vi "HumanDriveButtonBoxSourceClimbProcessor.vi"(6 "Processor":bool, 7 "Climb":bool, 8 "LeftSourceLeft":bool, 9 "LeftSourceRight":bool, 10 "RightSourceLeft":bool, 11 "RightSourceRight":bool) -> (3 "DriveTraj":bool)   [LabVIEW 2023]
uses:
  HumanGlobal.vi
  <vilib>/Rock Robotics/WPI/ThirdParty/JAS_Junk/TrajLib/Trajectory_Library.lvlib
  HumanBoxSourceClimbProcessorENUM.ctl
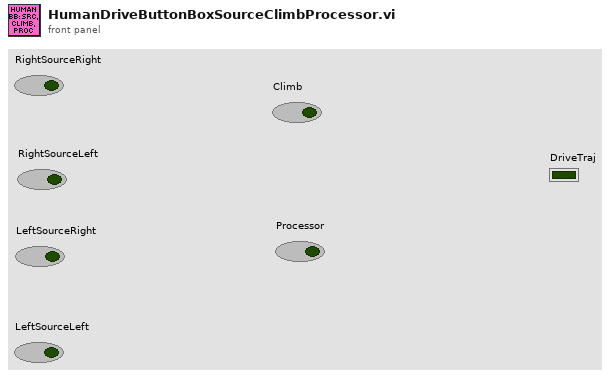
[diagram p1: front panel]
types:
  T1 = typedef "HumanBoxSourceClimbProcessorENUM.ctl" = enum16{"NoTraj", "RightSourceRight", "RightSourceLeft", "LeftSourceRight", "LeftSourceLeft", "Climb", "Processor"}
  T2 = typedef "WPI_DriverStationAllianceInfo.ctl" = enum16{"Red", "Blue", "Invalid"}
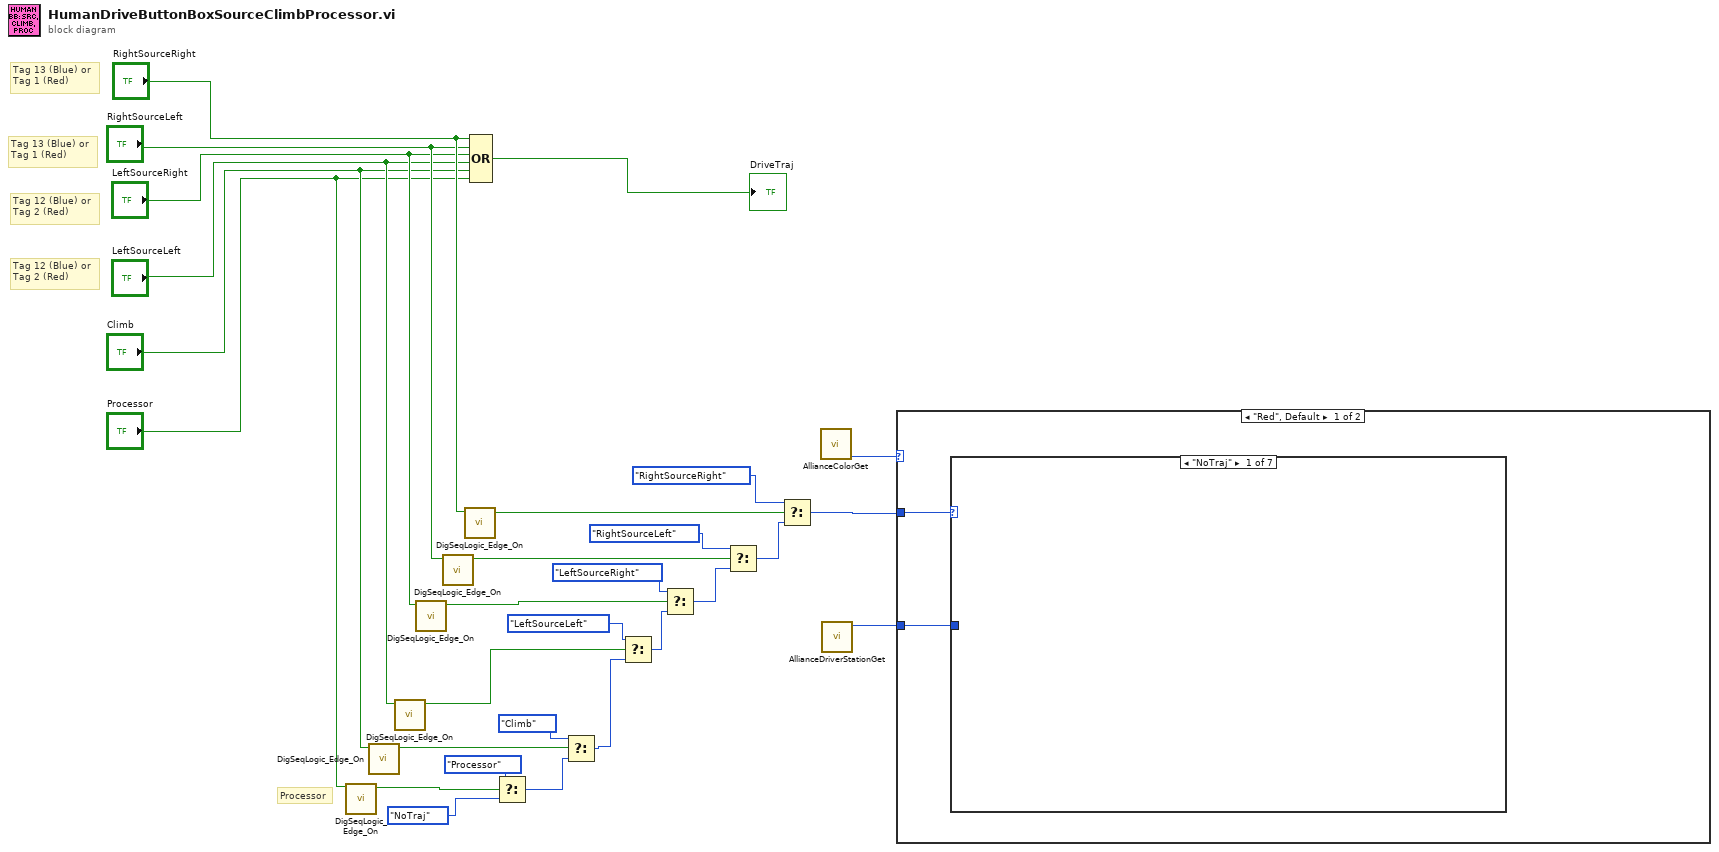
[diagram p0: block diagram]
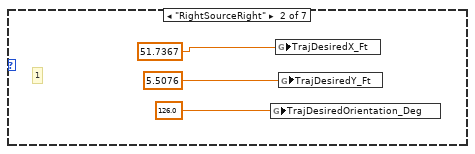
[diagram p2: hidden frame]
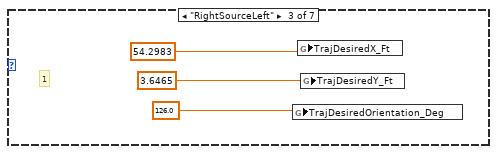
[diagram p3: hidden frame]
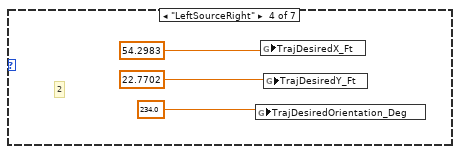
[diagram p4: hidden frame]
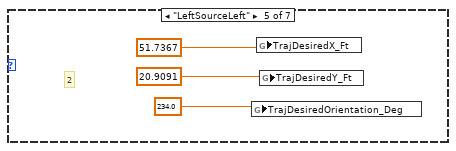
[diagram p5: hidden frame]
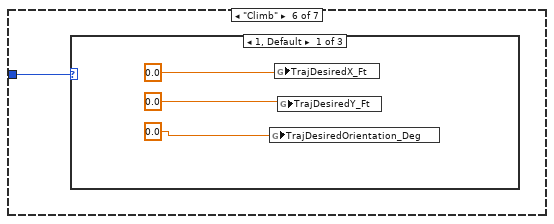
[diagram p6: hidden frame]
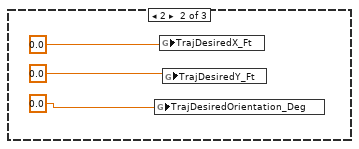
[diagram p7: hidden frame]
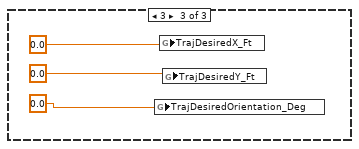
[diagram p8: hidden frame]
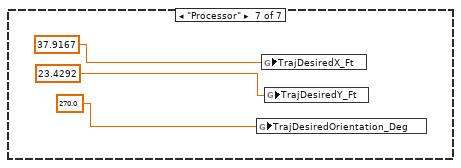
[diagram p9: hidden frame]
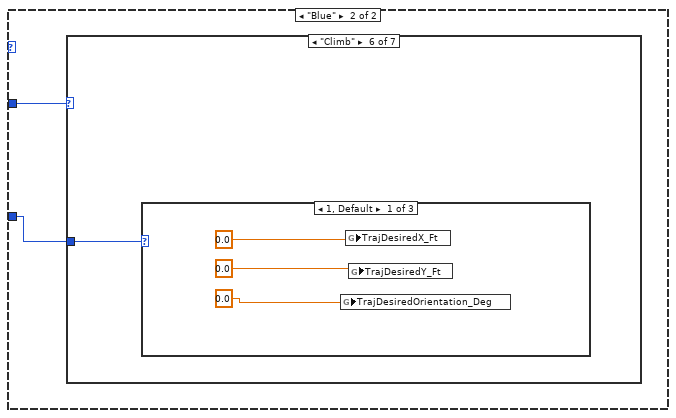
[diagram p10: hidden frame]
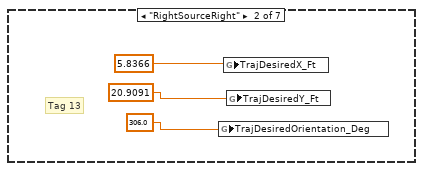
[diagram p12: hidden frame]
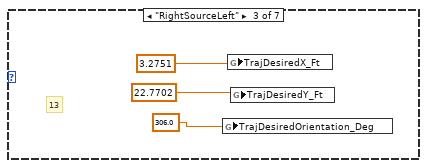
[diagram p13: hidden frame]
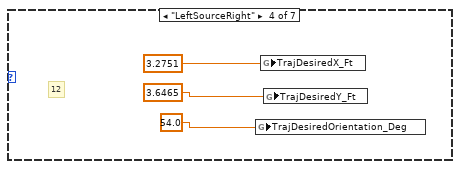
[diagram p14: hidden frame]
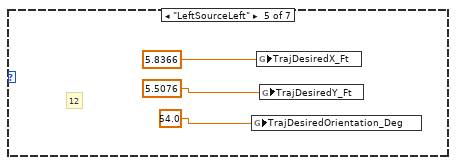
[diagram p15: hidden frame]
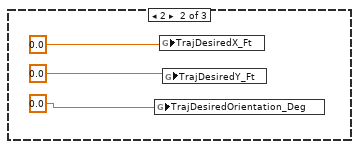
[diagram p16: hidden frame]
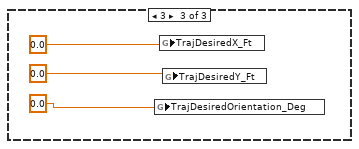
[diagram p17: hidden frame]
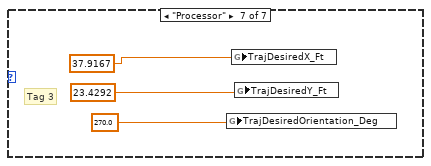
[diagram p18: hidden frame]
diagram:
  # "Tag 13 (Blue) or \nTag 1 (Red)"
  # "Tag 13 (Blue) or \nTag 1 (Red)"
  # "Tag 12 (Blue) or \nTag 2 (Red)"
  # "Tag 12 (Blue) or \nTag 2 (Red)"
  # "Processor"
  n1 = call <vilib>:"DigSeqLogic_Edge_On.vi"("Input"="Processor") -> ("On Edge"=w21:bool)  [unwired: 10 in]
  n2 = call <vilib>:"DigSeqLogic_Edge_On.vi"("Input"="Climb") -> ("On Edge"=w15:bool)  [unwired: 10 in]
  n3 = call <vilib>:"DigSeqLogic_Edge_On.vi"("Input"="LeftSourceLeft") -> ("On Edge"=w14:bool)  [unwired: 10 in]
  n4 = call <vilib>:"DigSeqLogic_Edge_On.vi"("Input"="LeftSourceRight") -> ("On Edge"=w13:bool)  [unwired: 10 in]
  n5 = call <vilib>:"DigSeqLogic_Edge_On.vi"("Input"="RightSourceLeft") -> ("On Edge"=w12:bool)  [unwired: 10 in]
  n6 = call <vilib>:"DigSeqLogic_Edge_On.vi"("Input"="RightSourceRight") -> ("On Edge"=w11:bool)  [unwired: 10 in]
  n7 = Compound Arithmetic op=OR("RightSourceRight", "RightSourceLeft", "LeftSourceRight", "LeftSourceLeft", "Climb", "Processor") -> (→"DriveTraj":bool)
  n8 = Select(t=HumanBoxSourceClimbProcessorENUM."Processor", s=w21, f=HumanBoxSourceClimbProcessorENUM."NoTraj") -> (s? t:f=w20:T1)
  n9 = Select(t=HumanBoxSourceClimbProcessorENUM."Climb", s=w15, f=w20) -> (s? t:f=w19:T1)
  n10 = Select(t=HumanBoxSourceClimbProcessorENUM."LeftSourceLeft", s=w14, f=w19) -> (s? t:f=w18:T1)
  n11 = Select(t=HumanBoxSourceClimbProcessorENUM."LeftSourceRight", s=w13, f=w18) -> (s? t:f=w17:T1)
  n12 = Select(t=HumanBoxSourceClimbProcessorENUM."RightSourceLeft", s=w12, f=w17) -> (s? t:f=w16:T1)
  n13 = Select(t=HumanBoxSourceClimbProcessorENUM."RightSourceRight", s=w11, f=w16) -> (s? t:f=w3:T1)
  n14 = call "AllianceColorGet.vi"() -> ("AllianceColor"=w2:T2)  [unwired: 11 in]
  n15 = call "AllianceDriverStationGet.vi"() -> ("Position"=w1:i32)  [unwired: 11 in]
  n16 = case shown="\"Red\", Default" w2 {
    tunnel: w3 -> [w30 w57]
    tunnel: w1 -> [w29 w56]
    frame "Red", Default {
      n17 = case shown="\"NoTraj\"" w30 {
        tunnel: w29 -> [_ _ _ _ _ w43 _]
        frame "NoTraj" {
        }
        frame "RightSourceRight" {
          # "1"
          n18 = global write "HumanGlobal.vi" "TrajDesiredOrientation_Deg"(126.0 ("TrajDesiredOrientation_Deg")) -> ()
          n19 = global write "HumanGlobal.vi" "TrajDesiredX_Ft"(51.7367 ("TrajDesiredX_Ft")) -> ()
          n20 = global write "HumanGlobal.vi" "TrajDesiredY_Ft"(5.5076 ("TrajDesiredY_Ft")) -> ()
        }
        frame "RightSourceLeft" {
          # "1"
          n21 = global write "HumanGlobal.vi" "TrajDesiredOrientation_Deg"(126.0 ("TrajDesiredOrientation_Deg")) -> ()
          n22 = global write "HumanGlobal.vi" "TrajDesiredX_Ft"(54.2983 ("TrajDesiredX_Ft")) -> ()
          n23 = global write "HumanGlobal.vi" "TrajDesiredY_Ft"(3.6465 ("TrajDesiredY_Ft")) -> ()
        }
        frame "LeftSourceRight" {
          # "2"
          n24 = global write "HumanGlobal.vi" "TrajDesiredOrientation_Deg"(234.0 ("TrajDesiredOrientation_Deg")) -> ()
          n25 = global write "HumanGlobal.vi" "TrajDesiredX_Ft"(54.2983 ("TrajDesiredX_Ft")) -> ()
          n26 = global write "HumanGlobal.vi" "TrajDesiredY_Ft"(22.7702 ("TrajDesiredY_Ft")) -> ()
        }
        frame "LeftSourceLeft" {
          # "2"
          n27 = global write "HumanGlobal.vi" "TrajDesiredOrientation_Deg"(234.0 ("TrajDesiredOrientation_Deg")) -> ()
          n28 = global write "HumanGlobal.vi" "TrajDesiredX_Ft"(51.7367 ("TrajDesiredX_Ft")) -> ()
          n29 = global write "HumanGlobal.vi" "TrajDesiredY_Ft"(20.9091 ("TrajDesiredY_Ft")) -> ()
        }
        frame "Climb" {
          n30 = case shown="1, Default" w43 {
            frame 1, Default {
              n31 = global write "HumanGlobal.vi" "TrajDesiredOrientation_Deg"(0.0 ("TrajDesiredOrientation_Deg")) -> ()
              n32 = global write "HumanGlobal.vi" "TrajDesiredX_Ft"(0.0 ("TrajDesiredX_Ft")) -> ()
              n33 = global write "HumanGlobal.vi" "TrajDesiredY_Ft"(0.0 ("TrajDesiredY_Ft")) -> ()
            }
            frame 2 {
              n34 = global write "HumanGlobal.vi" "TrajDesiredOrientation_Deg"(0.0 ("TrajDesiredOrientation_Deg")) -> ()
              n35 = global write "HumanGlobal.vi" "TrajDesiredX_Ft"(0.0 ("TrajDesiredX_Ft")) -> ()
              n36 = global write "HumanGlobal.vi" "TrajDesiredY_Ft"(0.0 ("TrajDesiredY_Ft")) -> ()
            }
            frame 3 {
              n37 = global write "HumanGlobal.vi" "TrajDesiredOrientation_Deg"(0.0 ("TrajDesiredOrientation_Deg")) -> ()
              n38 = global write "HumanGlobal.vi" "TrajDesiredX_Ft"(0.0 ("TrajDesiredX_Ft")) -> ()
              n39 = global write "HumanGlobal.vi" "TrajDesiredY_Ft"(0.0 ("TrajDesiredY_Ft")) -> ()
            }
          }
        }
        frame "Processor" {
          n40 = global write "HumanGlobal.vi" "TrajDesiredOrientation_Deg"(270.0 ("TrajDesiredOrientation_Deg")) -> ()
          n41 = global write "HumanGlobal.vi" "TrajDesiredX_Ft"(37.9167 ("TrajDesiredX_Ft")) -> ()
          n42 = global write "HumanGlobal.vi" "TrajDesiredY_Ft"(23.4292 ("TrajDesiredY_Ft")) -> ()
        }
      }
    }
    frame "Blue" {
      n43 = case shown="\"Climb\"" w57 {
        tunnel: w56 -> [_ _ _ _ _ w70 _]
        frame "NoTraj" {
        }
        frame "RightSourceRight" {
          # "Tag 13"
          n44 = global write "HumanGlobal.vi" "TrajDesiredOrientation_Deg"(306.0 ("TrajDesiredOrientation_Deg")) -> ()
          n45 = global write "HumanGlobal.vi" "TrajDesiredX_Ft"(5.8366 ("TrajDesiredX_Ft")) -> ()
          n46 = global write "HumanGlobal.vi" "TrajDesiredY_Ft"(20.9091 ("TrajDesiredY_Ft")) -> ()
        }
        frame "RightSourceLeft" {
          # "13"
          n47 = global write "HumanGlobal.vi" "TrajDesiredOrientation_Deg"(306.0 ("TrajDesiredOrientation_Deg")) -> ()
          n48 = global write "HumanGlobal.vi" "TrajDesiredX_Ft"(3.2751 ("TrajDesiredX_Ft")) -> ()
          n49 = global write "HumanGlobal.vi" "TrajDesiredY_Ft"(22.7702 ("TrajDesiredY_Ft")) -> ()
        }
        frame "LeftSourceRight" {
          # "12"
          n50 = global write "HumanGlobal.vi" "TrajDesiredOrientation_Deg"(54.0 ("TrajDesiredOrientation_Deg")) -> ()
          n51 = global write "HumanGlobal.vi" "TrajDesiredX_Ft"(3.2751 ("TrajDesiredX_Ft")) -> ()
          n52 = global write "HumanGlobal.vi" "TrajDesiredY_Ft"(3.6465 ("TrajDesiredY_Ft")) -> ()
        }
        frame "LeftSourceLeft" {
          # "12"
          n53 = global write "HumanGlobal.vi" "TrajDesiredOrientation_Deg"(54.0 ("TrajDesiredOrientation_Deg")) -> ()
          n54 = global write "HumanGlobal.vi" "TrajDesiredX_Ft"(5.8366 ("TrajDesiredX_Ft")) -> ()
          n55 = global write "HumanGlobal.vi" "TrajDesiredY_Ft"(5.5076 ("TrajDesiredY_Ft")) -> ()
        }
        frame "Climb" {
          n56 = case shown="1, Default" w70 {
            frame 1, Default {
              n57 = global write "HumanGlobal.vi" "TrajDesiredOrientation_Deg"(0.0 ("TrajDesiredOrientation_Deg")) -> ()
              n58 = global write "HumanGlobal.vi" "TrajDesiredX_Ft"(0.0 ("TrajDesiredX_Ft")) -> ()
              n59 = global write "HumanGlobal.vi" "TrajDesiredY_Ft"(0.0 ("TrajDesiredY_Ft")) -> ()
            }
            frame 2 {
              n60 = global write "HumanGlobal.vi" "TrajDesiredOrientation_Deg"(0.0 ("TrajDesiredOrientation_Deg")) -> ()
              n61 = global write "HumanGlobal.vi" "TrajDesiredX_Ft"(0.0 ("TrajDesiredX_Ft")) -> ()
              n62 = global write "HumanGlobal.vi" "TrajDesiredY_Ft"(0.0 ("TrajDesiredY_Ft")) -> ()
            }
            frame 3 {
              n63 = global write "HumanGlobal.vi" "TrajDesiredOrientation_Deg"(0.0 ("TrajDesiredOrientation_Deg")) -> ()
              n64 = global write "HumanGlobal.vi" "TrajDesiredX_Ft"(0.0 ("TrajDesiredX_Ft")) -> ()
              n65 = global write "HumanGlobal.vi" "TrajDesiredY_Ft"(0.0 ("TrajDesiredY_Ft")) -> ()
            }
          }
        }
        frame "Processor" {
          # "Tag 3"
          n66 = global write "HumanGlobal.vi" "TrajDesiredOrientation_Deg"(270.0 ("TrajDesiredOrientation_Deg")) -> ()
          n67 = global write "HumanGlobal.vi" "TrajDesiredX_Ft"(37.9167 ("TrajDesiredX_Ft")) -> ()
          n68 = global write "HumanGlobal.vi" "TrajDesiredY_Ft"(23.4292 ("TrajDesiredY_Ft")) -> ()
        }
      }
    }
  }
